vi "getWfFromFile.vi"(8 "error in (no error)":errorcluster, 9 "Sensor Name":string[](array[string])=["R:4,4 S:0,0", "R:0,4 S:2,0", "R:0,0 S:2,2", "R:4,0 S:0,2"], 10 "Wfs Err Data":path=path "/home/ttsai/Documents/stash/ts_tcs_ofc/testData/lsst_wfs_error_iter0.z4c", 11 "OptStateEsti in":refnum<class "OptStateEsti.lvclass">) -> (0 "error out":errorcluster, 1 "Field Idx":i32[](array[numeric]), 2 "Wavefront Error":dbl[][](array[numeric]), 3 "OptStateEsti out":refnum<class "OptStateEsti.lvclass">)   [LabVIEW 2016, in "OfcFunc.lvlib" / "OptStateEsti.lvclass"]
doc: "Get the wavefront error from the file."
uses:
  OptStateEsti.lvclass
  MatOper/MatOper.lvclass
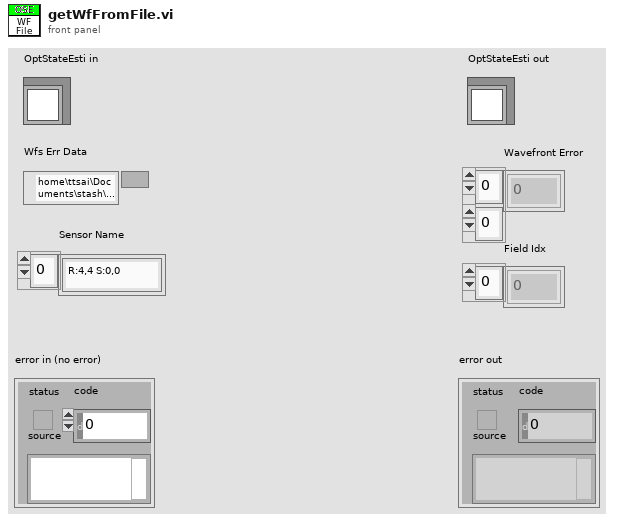
[diagram p1: front panel]
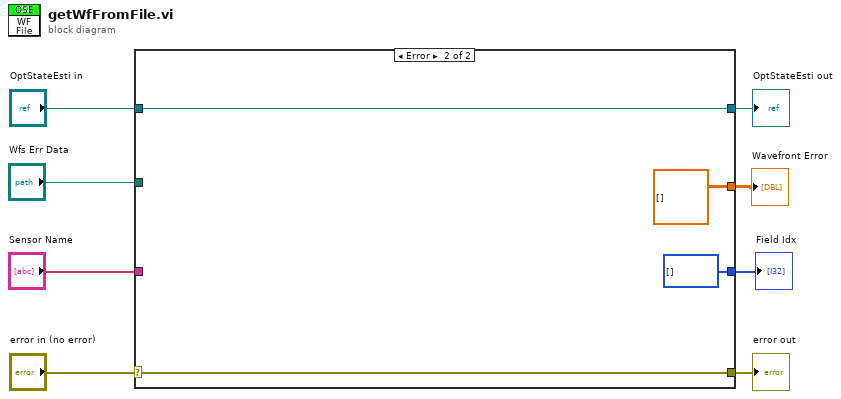
[diagram p0: block diagram]
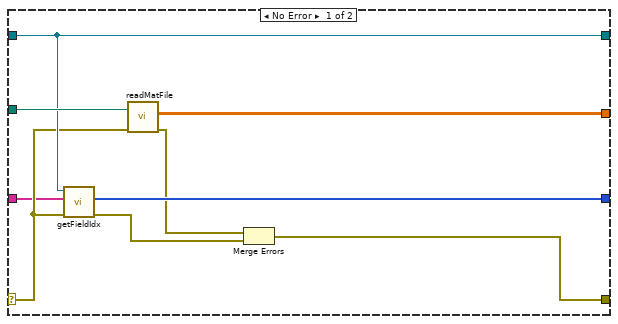
[diagram p2: hidden frame]
diagram:
  n1 = case shown="Error" "error in (no error)" {
    selector: "error in (no error)" -> [w13 w21]
    tunnel: [w10 w21] -> w7
    tunnel: [w15 w20] -> w5
    tunnel: "OptStateEsti in" -> [w15 w20]
    tunnel: "Wfs Err Data" -> [w17 _]
    tunnel: [w16 dbl[][] [] ("Matrix")] -> w3
    tunnel: [w14 i32[] [] ("Field Idx")] -> w2
    tunnel: "Sensor Name" -> [w9 _]
    frame No Error {
      n2 = call "getFieldIdx.vi"("error in (no error)"=w13, "Sensor Name"=w9, "OptStateEsti in"=w15) -> ("error out"=w12:errorcluster, "Field Idx"=w14:i32[])  [unwired: 6 in, 1 out]
      n3 = call "readMatFile.vi"("Path"=w17, "error in (no error)"=w13) -> ("error out"=w11:errorcluster, "Matrix"=w16:dbl[][])  [unwired: 7 in, 1 out]
      n4 = Merge Errors(w11, w12) -> (w10:errorcluster)
    }
    frame Error {
    }
  }
  "error out" <- w7
  "OptStateEsti out" <- w5
  "Wavefront Error" <- w3
  "Field Idx" <- w2
